vi "14.2 Rotate Detect-1.vi"(8 "ErrI":errorcluster) -> ()   [LabVIEW 2016]
uses:
  <vilib>/vision/Image Controls.llb/IMAQ Image.ctl
  <vilib>/vision/NI_Vision_Development_Module.lvlib
panel:
  out "Tmplate":T1(plugin-control)
  out "Center":cluster{"X":sgl, "Y":sgl} {"X" format="%#_3g"; "Y" format="%#_3g"}
  out "Degree:":sgl format="%#_4g"
  out "Points":cluster{"X":sgl, "Y":sgl}[](array[cluster]) {"X" format="%#_3g"; "Y" format="%#_3g"}
  out "IMG":T1(plugin-control)
  in  "Next":bool
  in  "Exit":bool
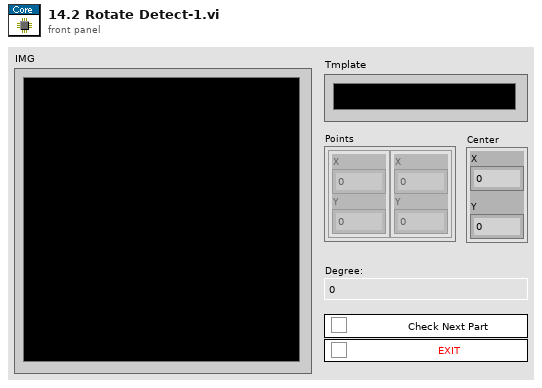
[diagram p1: front panel]
types:
  T1 = typedef "IMAQ Image.ctl" = refnum<image>
  T2 = cluster{"Number of Matches Requested":i32, "Minimum Match Score":sgl, "Angle Ranges":cluster{"Start Angle":sgl, "End Angle":sgl}[]}
  T3 = cluster{"Tmp":T1, "Src":T1, "Dst":T1, "Parts":string[], "Center":cluster{"X":sgl, "Y":sgl}}
  T4 = typedef "Image Type" = u32
  T5 = typedef "IMAQ Circle" = cluster{"Center X":i32, "Center Y":i32, "Inner Radius":i32, "Outer Radius":i32, "Start Angle":dbl, "End Angle":dbl}
  T6 = typedef "ROI Descriptor" = cluster{"Global Rectangle":i32[], "Contours":cluster{"ID":enum32{"External", "Internal"}, "Type":u32, "Coordinates":i32[]}[]}
  T7 = cluster{"Center (Pixels)":cluster{"X":sgl, "Y":sgl}, "Radius (Pixels)":dbl, "Center (Real-World)":cluster{"X":sgl, "Y":sgl}, "Radius (Real-World)":dbl, "Roundness (Real-World)":dbl, "Average Strength":dbl, "Average SNR (dB)":dbl}
  T8 = cluster{"Position":cluster{"x":sgl, "y":sgl}, "Angle":sgl, "Scale":sgl, "Score":sgl, "Bounding Box":cluster{"x":sgl, "y":sgl}[]}[]
  T9 = cluster{"Position":cluster{"x":sgl, "y":sgl}, "Angle":sgl, "Scale":sgl, "Score":sgl, "Bounding Box":cluster{"x":sgl, "y":sgl}[]}
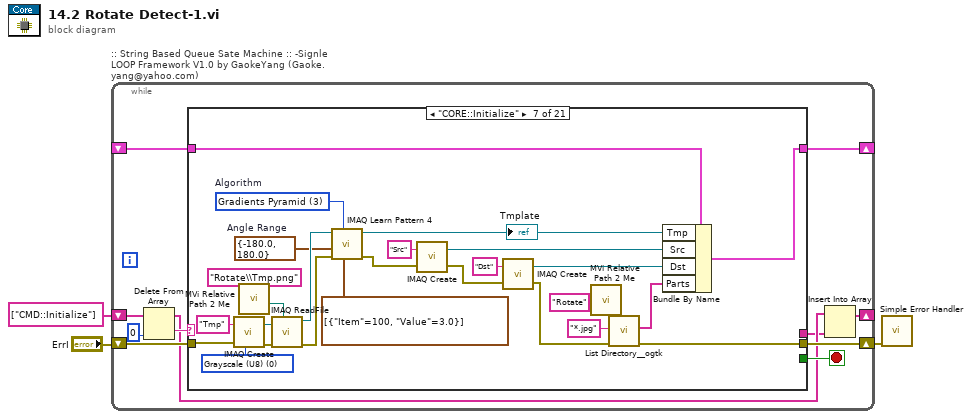
[diagram p0: block diagram]
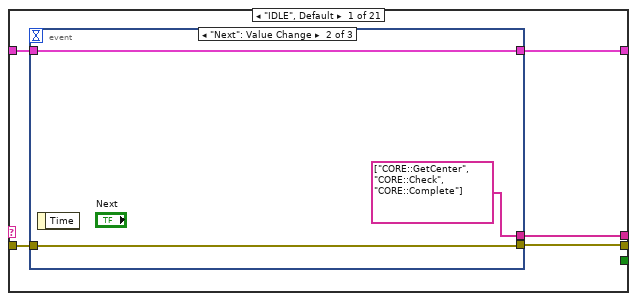
[diagram p2: hidden frame]
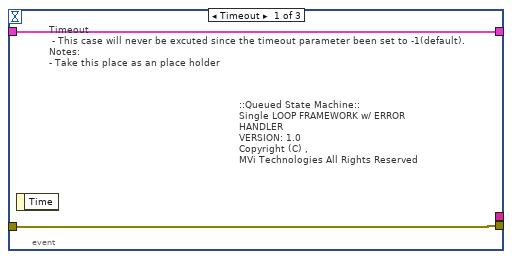
[diagram p3: hidden frame]
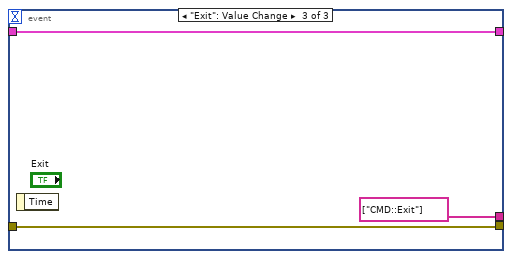
[diagram p4: hidden frame]
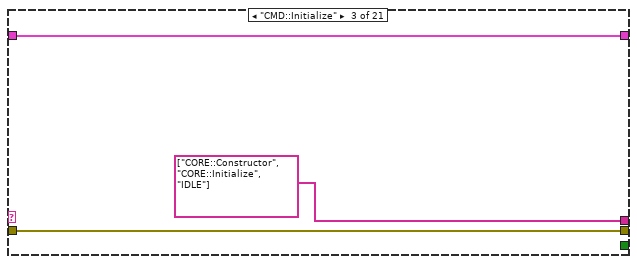
[diagram p6: hidden frame]
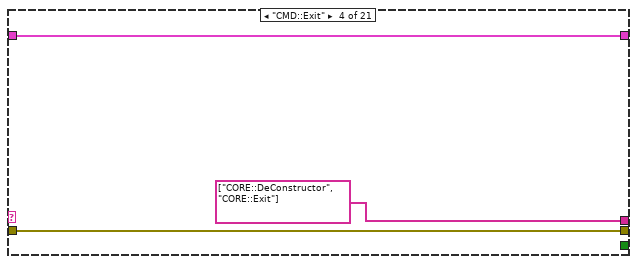
[diagram p7: hidden frame]
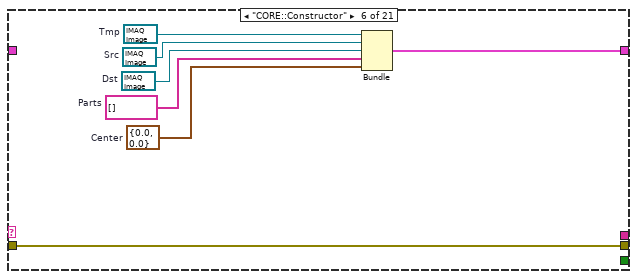
[diagram p9: hidden frame]
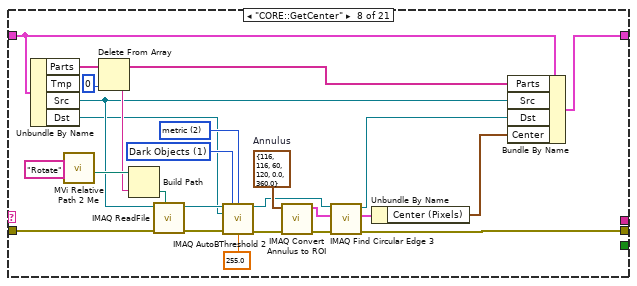
[diagram p10: hidden frame]
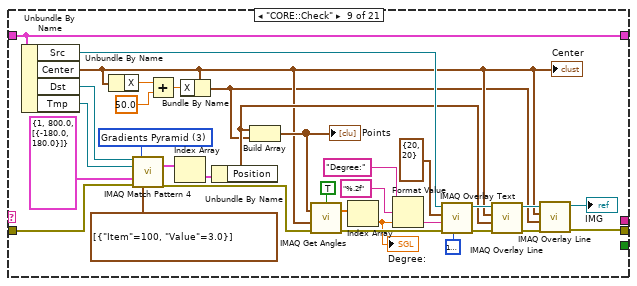
[diagram p11: hidden frame]
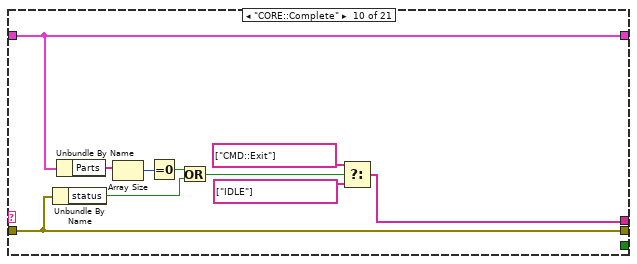
[diagram p12: hidden frame]
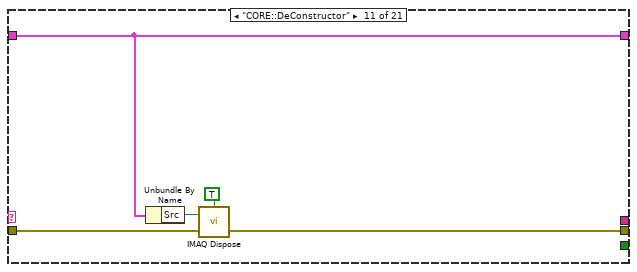
[diagram p13: hidden frame]
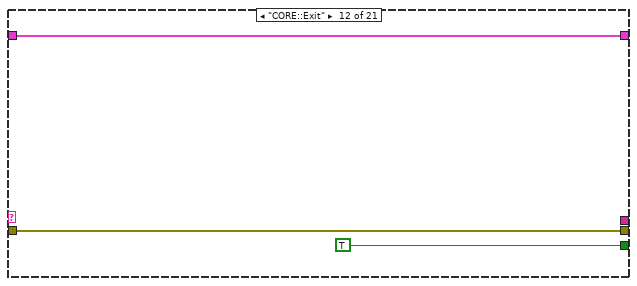
[diagram p14: hidden frame]
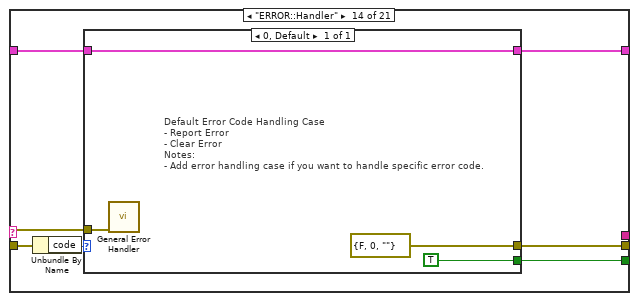
[diagram p16: hidden frame]
diagram:
  n1 = while ":: String Based Queue Sate Machine :: -Signle LOOP Framework V1.0 by GaokeYang (Gaoke.yang@yahoo.com)" {
    shift-right: [w11] -> w1
    shift-left: "ErrI" -> [w9]
    shift-right: [w13] -> _
    shift-left: _ -> [w12]
    shift-right: [w4] -> _
    shift-left: string[] ["CMD::Initialize"] -> [w10]
    stop <- w14 stop-if-true
    n2 = Delete From Array(array=w10, index=0) -> (deleted portion=w8:string, array with subset deleted=w6:string[])  [unwired: 1 in]
    n3 = case shown="\"CORE::Initialize\"" w8 {
      tunnel: [w18 w29 w31 w34 w37 w43 w62 w87 w100 w136 w144 w146 w150 w153 w161 w163 w165 w168 w170 w172 w173] -> w11
      tunnel: [_ _ _ _ _ _ _ _ _ _ _ TRUE _ w152 _ _ _ _ _ _ _] -> w14
      tunnel: w9 -> [w19 w29 w31 w34 w37 w43 w66 w92 w127 w136 w145 w146 w150 w151 w161 w163 w165 w168 w170 w172 w173]
      tunnel: [w16 w28 w32 w35 w36 w44 w69 w89 w130 w137 w143 w147 w149 w154 w162 w164 w166 w167 w169 w171 w174] -> w13
      tunnel: w12 -> [w17 w28 w32 w35 w36 _ w70 w90 w130 w137 w143 w147 w149 w155 w162 w164 w166 w167 w169 w171 w174]
      tunnel: [w15 _ string[] ["CORE::Constructor", "CORE::Initialize", "IDLE"] string[] ["CORE::DeConstructor", "CORE::Exit"] _ _ _ _ _ w138 _ _ _ _ _ _ _ _ _ _ _] -> w5
      frame "IDLE", Default {
        n4 = event shown="[1] \"Next\": Value Change" {
          selector: _ -> [_ _ _]
          dyn-events: _ -> [_ _ _]
          timeout: _ -> [_ _ _]
          tunnel: [w21 w24 w27] -> w18
          tunnel: w19 -> [w21 w24 w27]
          tunnel: [w20 w23 w26] -> w16
          tunnel: w17 -> [w20 w23 w26]
          tunnel: [_ string[] ["CORE::GetCenter", "CORE::Check", "CORE::Complete"] string[] ["CMD::Exit"]] -> w15
          event Timeout {
            # "Timeout\n - This case will never be excuted since the timeout parameter been set to -1(default).\nNotes:\n- Take this place as an place holder"
            # "::Queued State Machine::\nSingle LOOP FRAMEWORK w/ ERROR HANDLER\nVERSION: 1.0\nCopyright (C) ,\nMVi Technologies All Rights Reserved"
            n5 = event-data() -> ()  [unwired: 1 in, 1 out]
          }
          event "Next": Value Change {
            n6 = event-data() -> ()  [unwired: 1 in, 1 out]
          }
          event "Exit": Value Change {
            n7 = event-data() -> ()  [unwired: 1 in, 1 out]
          }
        }
      }
      frame "-------- Commands ---------" {
      }
      frame "CMD::Initialize" {
      }
      frame "CMD::Exit" {
      }
      frame "------------ Core ------------" {
      }
      frame "CORE::Constructor" {
        w38 = cluster{"X":sgl, "Y":sgl} {"X"=0.0, "Y"=0.0}  # Center
        w39 = T1 refnum  # Dst
        w41 = T1 refnum  # Src
        w40 = string[] []  # Parts
        w42 = T1 refnum  # Tmp
        n8 = Bundle("Tmp"=w42, "Src"=w41, "Dst"=w39, "Parts"=w40, "Center"=w38) -> (w44:T3)  [unwired: 1 in]
      }
      frame "CORE::Initialize" {
        w46 = T4 0 items=["Grayscale (U8)", "Grayscale (I16)", "Grayscale (SGL)", "Complex (CSG)", "RGB (U32)", "HSL (U32)", "RGB (U64)", "Grayscale (U16)"] ("Image Type")
        w47 = cluster{"Start Angle":sgl, "End Angle":sgl} {"Start Angle"=-180.0, "End Angle"=180.0}  # Angle Range
        w48 = 3 items=["All", "Low Discrepancy Sampling", "Grayscale Value Pyramid", "Gradients Pyramid"]  # Algorithm
        n9 = call "IMAQ Create"("Image Name"="Tmp", "Image Type"=w46, "error in (no error)"=w66) -> ("Src"=w68:T1, "error out"=w67:errorcluster)  [unwired: 2 in]
        n10 = call "MVi Relative Path 2 Me.vi"("Relative Path"="Rotate\\Tmp.png" ("name or relative path")) -> ("Appended Dir"=w59:path)  [unwired: 5 in, 1 out]
        n11 = call "IMAQ ReadFile"("File Path"=w59, "error in (no error)"=w67, "Image"=w68) -> ("error out"=w52:errorcluster, "Image Out"=w50:T1)  [unwired: 4 in, 3 out]
        n12 = call "IMAQ Learn Pattern 4"("Advanced Options"=cluster{"Item":u16, "Value":dbl}[] [{"Item"=100, "Value"=3.0}], "Algorithm"=w48, "error in (no error)"=w52, "Angle Range"=w47, "Image"=w50) -> ("error out"=w51:errorcluster, "Template Image Out"=w45:T1)  [unwired: 4 in, 1 out]
        "Tmplate" <- w45
        n13 = call "IMAQ Create"("Image Name"="Src", "error in (no error)"=w51) -> ("Src"=w58:T1, "error out"=w56:errorcluster)  [unwired: 3 in]
        n14 = call "IMAQ Create"("Image Name"="Dst", "error in (no error)"=w56) -> ("Src"=w54:T1, "error out"=w53:errorcluster)  [unwired: 3 in]
        n15 = call "MVi Relative Path 2 Me.vi"("Relative Path"="Rotate" ("name or relative path")) -> ("Appended Dir"=w64:path)  [unwired: 5 in, 1 out]
        n16 = call "List Directory__ogtk.vi"("error in (no error)"=w53, "pattern"="*.jpg", "directory path"=w64) -> ("error out"=w62:errorcluster, "file names"=w55:string[])  [unwired: 1 in, 2 out]
        n17 = Bundle By Name(cluster=w70, "Tmp"=w45, "Src"=w58, "Dst"=w54, "Parts"=w55) -> (w69:T3)
      }
      frame "CORE::GetCenter" {
        w80 = T5 {"Center X"=116, "Center Y"=116, "Inner Radius"=60, "Outer Radius"=120, "Start Angle"=0.0, "End Angle"=360.0}  # Annulus
        w83 = u32 1 items=["Bright Objects", "Dark Objects"] ("Look For (Bright Objects)")
        w86 = 2 items=["clustering", "entropy", "metric", "moments", "inter-class variance"] ("Method (clustering)")
        n18 = Unbundle By Name(w90) -> ("Parts"=w88:string[], "Src"=w73:T1, "Dst"=w72:T1)  [unwired: 1 out]
        n19 = call "MVi Relative Path 2 Me.vi"("Relative Path"="Rotate" ("name or relative path")) -> ("Appended Dir"=w96:path)  [unwired: 5 in, 1 out]
        n20 = Delete From Array(array=w88, index=0) -> (deleted portion=w94:string, array with subset deleted=w91:string[])  [unwired: 1 in]
        n21 = Build Path(base path=w96, name or relative path=w94) -> (appended path=w93:path)
        n22 = call "IMAQ ReadFile"("File Path"=w93, "error in (no error)"=w92, "Image"=w73) -> ("error out"=w85:errorcluster, "Image Out"=w84:T1)  [unwired: 4 in, 3 out]
        n23 = call "IMAQ AutoBThreshold 2"("Image Src"=w84, "Look For (Bright Objects)"=w83, "Method (clustering)"=w86, "Image Dst"=w72, "error in (no error)"=w85, "Replace Value (1)"=sgl 255.0) -> ("Image Dst Out"=w76:T1, "error out"=w82:errorcluster)  [unwired: 7 in, 1 out]
        n24 = call "IMAQ Convert Annulus to ROI"("error in (no error)"=w82, "Annulus"=w80) -> ("error out"=w81:errorcluster, "ROI Descriptor"=w79:T6)  [unwired: 7 in]
        n25 = call "IMAQ Find Circular Edge 3"("error in (no error)"=w81, "ROI Descriptor"=w79, "Image"=w76) -> ("error out"=w87:errorcluster, "Fitted Circle"=w78:T7, "Image Out"=w75:T1)  [unwired: 4 in, 2 out]
        n26 = Unbundle By Name(w78) -> ("Center (Pixels)"=w77:cluster{"X":sgl, "Y":sgl})
        n27 = Bundle By Name(cluster=w90, "Parts"=w91, "Src"=w73, "Dst"=w75, "Center"=w77) -> (w89:T3)
      }
      frame "CORE::Check" {
        w124 = 3 items=["All", "Low Discrepancy Sampling", "Grayscale Value Pyramid", "Gradients Pyramid"] ("Algorithm")
        n28 = Unbundle By Name(w130) -> ("Src"=w108:T1, "Center"=w99:cluster{"X":sgl, "Y":sgl}, "Dst"=w126:T1, "Tmp"=w125:T1)
        "Center" <- w99
        n29 = Unbundle By Name(w99) -> ("X"=w117:sgl)
        n30 = call "IMAQ Match Pattern 4"("Image"=w126, "Algorithm"=w124, "Template Image"=w125, "Parameters"=T2 {"Number of Matches Requested"=1, "Minimum Match Score"=800.0, "Angle Ranges"=[{"Start Angle"=-180.0, "End Angle"=180.0}]}, "error in (no error)"=w127, "Advanced Options"=cluster{"Item":u16, "Value":dbl}[] [{"Item"=100, "Value"=3.0}]) -> ("Matches (pixel)"=w121:T8, "error out"=w119:errorcluster)  [unwired: 5 in, 3 out]
        n31 = Add(x=w117, y=sgl 50.0) -> (x+y=w115:sgl)
        n32 = Index Array(array=w121) -> (element=w120:T9)  [unwired: 1 in]
        n33 = Bundle By Name(cluster=w99, "X"=w115) -> (w98:cluster{"X":sgl, "Y":sgl})
        n34 = Unbundle By Name(w120) -> ("Position"=w104:cluster{"x":sgl, "y":sgl})
        n35 = Build Array(w104, w98) -> (w114:cluster{"X":sgl, "Y":sgl}[])
        "Points" <- w114
        n36 = call "IMAQ Get Angles"("error in (no error)"=w119, "Vertex"=w99, "Points"=w114, "Use Vertex (No)"=TRUE) -> ("error out"=w118:errorcluster, "Angles (deg)"=w112:sgl[])  [unwired: 1 in, 1 out]
        n37 = Index Array(array=w112) -> (element=w113:sgl)  [unwired: 1 in]
        "Degree:" <- w113
        n38 = Format Value(string ("")="Degree:", format string="%.2f", value (0)=w113) -> (output string=w109:string)
        n39 = call "IMAQ Overlay Text"("Text Color (black)"=u32 16777224, "error in (no error)"=w118, "String"=w109, "Origin"=cluster{"X":i32, "Y":i32} {"X"=20, "Y"=20}, "Image"=w108) -> ("error out"=w106:errorcluster, "Image Out"=w105:T1)  [unwired: 5 in]
        n40 = call "IMAQ Overlay Line"("error in (no error)"=w106, "End Point"=w104, "Start Point"=w99, "Image"=w105) -> ("error out"=w103:errorcluster, "Image Out"=w102:T1)  [unwired: 6 in]
        n41 = call "IMAQ Overlay Line"("error in (no error)"=w103, "End Point"=w98, "Start Point"=w99, "Image"=w102) -> ("error out"=w100:errorcluster, "Image Out"=→"IMG":T1)  [unwired: 6 in]
      }
      frame "CORE::Complete" {
        n42 = Unbundle By Name(w136) -> ("status"=w132:bool)
        n43 = Unbundle By Name(w137) -> ("Parts"=w135:string[])
        n44 = Array Size(array=w135) -> (size(s)=w134:i32)
        n45 = Equal To 0?(x=w134) -> (x = 0?=w133:bool)
        n46 = Or(x=w133, y=w132) -> (x .or. y?=w131:bool)
        n47 = Select(t=string[] ["CMD::Exit"], s=w131, f=string[] ["IDLE"]) -> (s? t:f=w138:string[])
      }
      frame "CORE::DeConstructor" {
        n48 = Unbundle By Name(w143) -> ("Src"=w142:T1)
        n49 = call "IMAQ Dispose"("All Images? (No)"=TRUE, "Image"=w142, "error in (no error)"=w145) -> ("error out"=w144:errorcluster)  [unwired: 3 in]
      }
      frame "CORE::Exit" {
      }
      frame "-------- Error Handle--------" {
      }
      frame "ERROR::Handler" {
        n50 = Unbundle By Name(w151) -> ("code"=w156:i32)
        n51 = case shown="0, Default" w156 {
          tunnel: [w160] -> w154
          tunnel: w155 -> [w160]
          tunnel: [errorcluster {"status"=FALSE, "code"=0, "source"=""} ("error out")] -> w153
          tunnel: [TRUE] -> w152
          tunnel: w151 -> [w158]
          frame 0, Default {
            # "Default Error Code Handling Case\n- Report Error\n- Clear Error \nNotes:\n- Add error handling case if you want to handle specific error code."
            n52 = call <vilib>:"General Error Handler.vi"("error in (no error)"=w158) -> ()  [unwired: 10 in, 5 out]
          }
        }
      }
      frame "------------  GUI  ------------" {
      }
      frame "GUI::Initialize" {
      }
      frame "GUI::SetCusor" {
      }
      frame "GUI::SetMenu" {
      }
      frame "------------ USER -----------" {
      }
      frame "USER::Case1" {
      }
      frame "USER::Case2" {
      }
    }
    n53 = Insert Into Array(array=w6, new element=w5) -> (w4:string[])  [unwired: 1 in]
  }
  n54 = call <vilib>:"Simple Error Handler.vi"("error in (no error)"=w1) -> ()  [unwired: 4 in, 5 out]
